vi "percentage.vi"(1 "max range":dbl, 2 "data read":dbl, 3 "minimum value":dbl, 4 "maximum value":dbl) -> (0 "percentage of mac range":dbl)   [LabVIEW 2023]
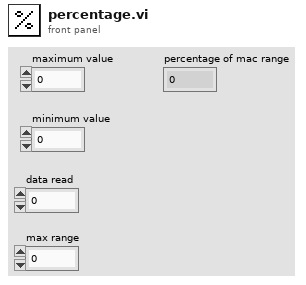
[diagram p1: front panel]
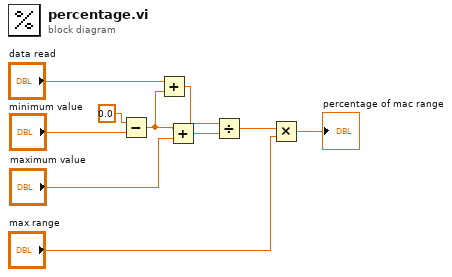
[diagram p0: block diagram]
diagram:
  n1 = Subtract(x=0.0, y="minimum value") -> (x-y=w5:dbl)
  n2 = Add(x="data read", y=w5) -> (x+y=w8:dbl)
  n3 = Add(x=w5, y="maximum value") -> (x+y=w9:dbl)
  n4 = Divide(x=w8, y=w9) -> (x/y=w3:dbl)
  n5 = Multiply(x=w3, y="max range") -> (x*y=→"percentage of mac range":dbl)
